vi "05.1 Writing Delimited Configuration Files.vi"() -> ()   [LabVIEW 2019]
uses:
  <vilib>/Utility/file.llb/Write Delimited Spreadsheet (string).vi
  <vilib>/Utility/file.llb/Read Delimited Spreadsheet (string).vi
panel:
  out "Found?":bool
  in  "Key":string
  out "value":string
  out "AO Channel":string
  out "AI Channel":string
  out "Samples per Channel":i32
  out "Sample Rate":dbl
  out "Error Out":errorcluster
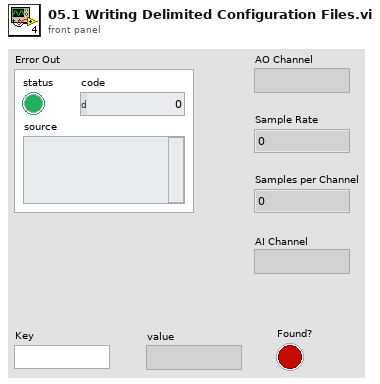
[diagram p1: front panel]
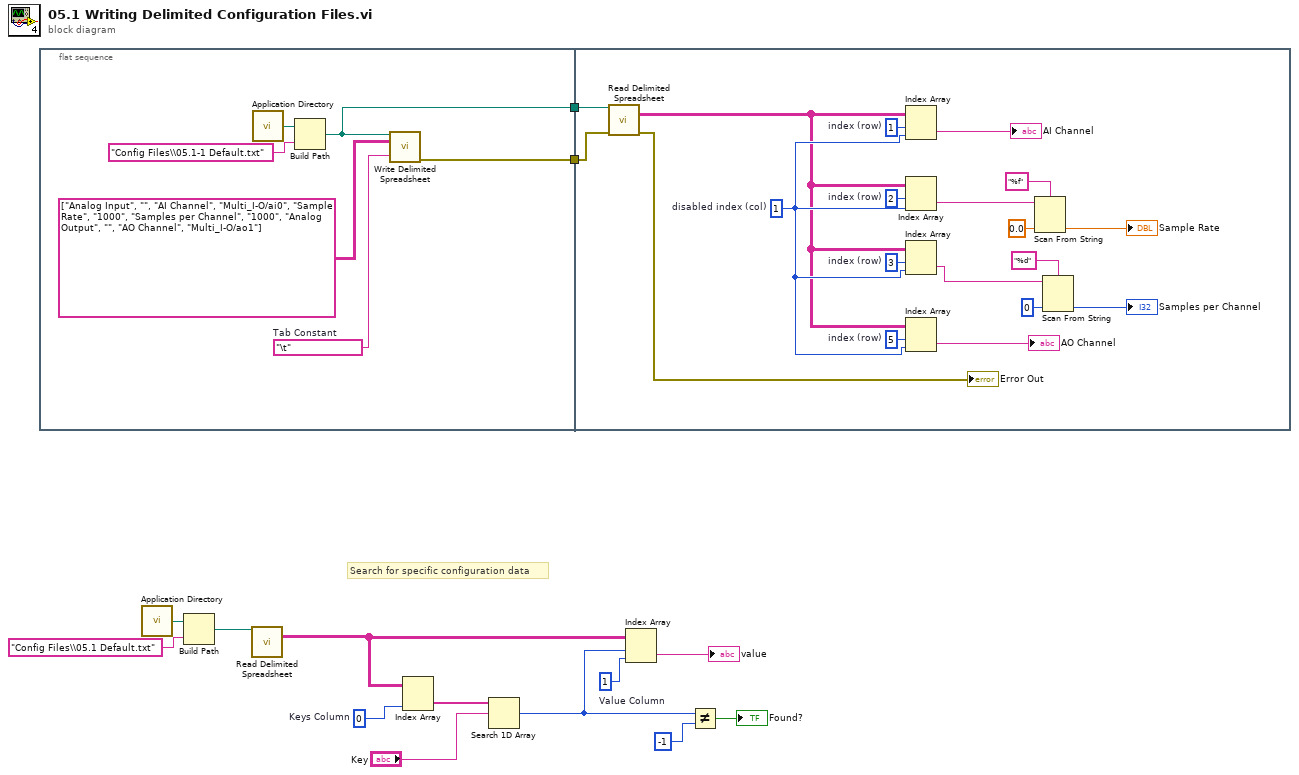
[diagram p0: block diagram]
diagram:
  w6 = 1  # Value Column
  w9 = 0  # Keys Column
  # "Search for specific configuration data"
  n1 = flat-sequence {
    tunnel: [w16] -> w14
    tunnel: [w15] -> w13
    tunnel: w14 -> [w39]
    tunnel: w13 -> [w38]
    frame #0 {
      w17 = "\t"  # Tab Constant
      n2 = call <vilib>:"Application Directory.vi"() -> ("Application Directory"=w20:path)
      n3 = Build Path(base path=w20, name or relative path="Config Files\\05.1-1 Default.txt") -> (appended path=w16:path)
      n4 = call-poly <vilib>:"Write Delimited Spreadsheet.vi"("file path (dialog if empty)"=w16, "2D data"=string[][] [["Analog Input", ""], ["AI Channel", "Multi_I-O/ai0"], ["Sample Rate", "1000"], ["Samples per Channel", "1000"], ["Analog Output", ""], ["AO Channel", "Multi_I-O/ao1"]], "delimiter (\\t)"=w17) -> ("error out"=w15:errorcluster)  [unwired: 11 in, 1 out]
    }
    frame #1 {
      w25 = 5  # index (row)
      w24 = 1  # disabled index (col)
      w34 = 3  # index (row)
      w35 = 2  # index (row)
      w37 = 1  # index (row)
      n5 = call-poly <vilib>:"Read Delimited Spreadsheet.vi"("file path (dialog if empty)"=w39, "error in (no error)"=w38) -> ("all rows"=w21:string[][], "error out"=→"Error Out":errorcluster)  [unwired: 8 in, 4 out]
      n6 = Index Array "Index Array"(array=w21, index (row)=w37, index (col)=w24) -> (element=→"AI Channel":string)
      n7 = Index Array "Index Array"(array=w21, index (row)=w35, index (col)=w24) -> (element=w32:string)
      n8 = Index Array "Index Array"(array=w21, index (row)=w34, index (col)=w24) -> (element=w27:string)
      n9 = Index Array "Index Array"(array=w21, index (row)=w25, index (col)=w24) -> (element=→"AO Channel":string)
      n10 = Scan From String "Scan From String"(format string="%f", input string=w32, default 1=0.0 ("default value 1")) -> (output 1=→"Sample Rate":dbl)  [unwired: 2 in, 3 out]
      n11 = Scan From String "Scan From String"(format string="%d", input string=w27, default 1=0 ("default value 1")) -> (output 1=→"Samples per Channel":i32)  [unwired: 2 in, 3 out]
    }
  }
  n12 = call <vilib>:"Application Directory.vi"() -> ("Application Directory"=w11:path)
  n13 = Build Path(base path=w11, name or relative path="Config Files\\05.1 Default.txt") -> (appended path=w10:path)
  n14 = call-poly <vilib>:"Read Delimited Spreadsheet.vi"("file path (dialog if empty)"=w10) -> ("all rows"=w8:string[][])  [unwired: 9 in, 5 out]
  n15 = Index Array "Index Array"(array=w8, index (col)=w9) -> (element=w7:string[])  [unwired: 1 in]
  n16 = Search 1D Array(1D array=w7, element="Key") -> (index of element=w3:i32)  [unwired: 1 in]
  n17 = Index Array "Index Array"(array=w8, index (row)=w3, index (col)=w6) -> (element=→"value":string)
  n18 = Not Equal?(x=w3, y=-1) -> (x != y?=→"Found?":bool)
